vi "WaitToCount.vi"(10 "Count":i32=10000, 11 "Boolean-01":bool) -> (2 "Boolean-01 Count":i32, 3 "Boolean-01-Indicator":bool)   [LabVIEW 2015]
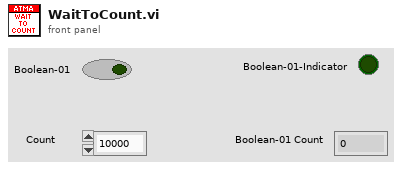
[diagram p1: front panel]
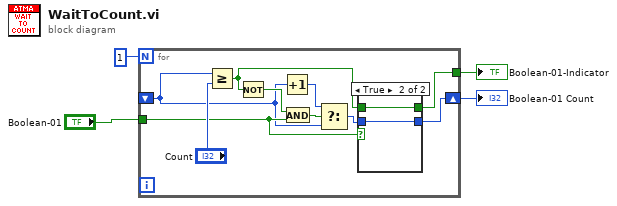
[diagram p0: block diagram]
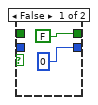
[diagram p2: hidden frame]
diagram:
  n1 = for {
    N: 1 -> [_]
    tunnel: "Boolean-01" -> [w12]
    shift-right: [w7] -> w2
    shift-left: _ -> [w10]
    tunnel: [w6] -> w1
    n2 = Greater Or Equal?(x=w10, y="Count") -> (x >= y?=w5:bool)
    n3 = Not(x=w5) -> (.not. x?=w13:bool)
    n4 = Increment(x=w10) -> (x+1=w9:i32)
    n5 = And(x=w13, y=w12) -> (x .and. y?=w11:bool)
    n6 = Select(t=w9, s=w11, f=w10) -> (s? t:f=w8:i32)
    n7 = case shown="True" w12 {
      tunnel: w8 -> [_ w18]
      tunnel: [0 w18] -> w7
      tunnel: [FALSE w17] -> w6
      tunnel: w5 -> [_ w17]
      frame False {
      }
      frame True {
      }
    }
  }
  "Boolean-01-Indicator" <- w1
  "Boolean-01 Count" <- w2
